vi "sutter_driver.vi"() -> ()   [LabVIEW 2016]
uses:
  <vilib>/Instr/_visa.llb/VISA Configure Serial Port (Instr).vi
panel:
  in  "Motor Poisition":dbl[][](array[numeric]) caption="Motor Poisition\nA               B"
  out "Position XYZ":dbl[](array[numeric])
  in  "Motor Select":u16(ring) items=["A"=1, "B"=2, "C"=3, "D"=4]
  in  "error in (no error)":errorcluster
  in  "stop":bool
  out "error out":errorcluster
  in  "VISA resource name":refnum<visa-resource-name>
  # "Motor Poisition\nA               B"
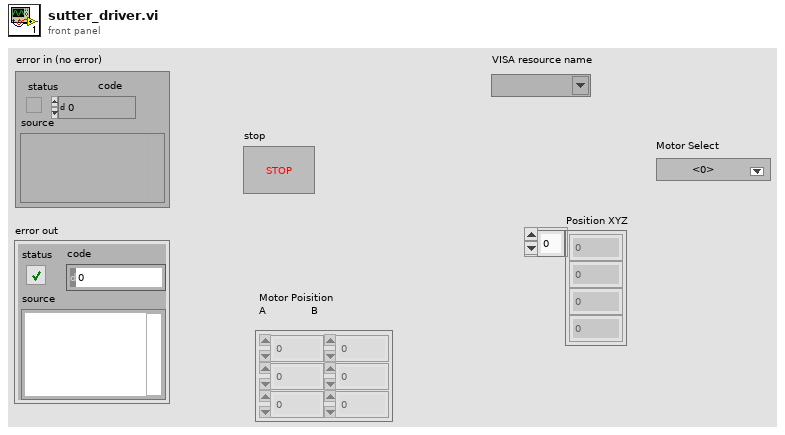
[diagram p1: front panel]
types:
  T1 = cluster{"Motor":u16, "Go Home":bool, "Position":dbl[]}
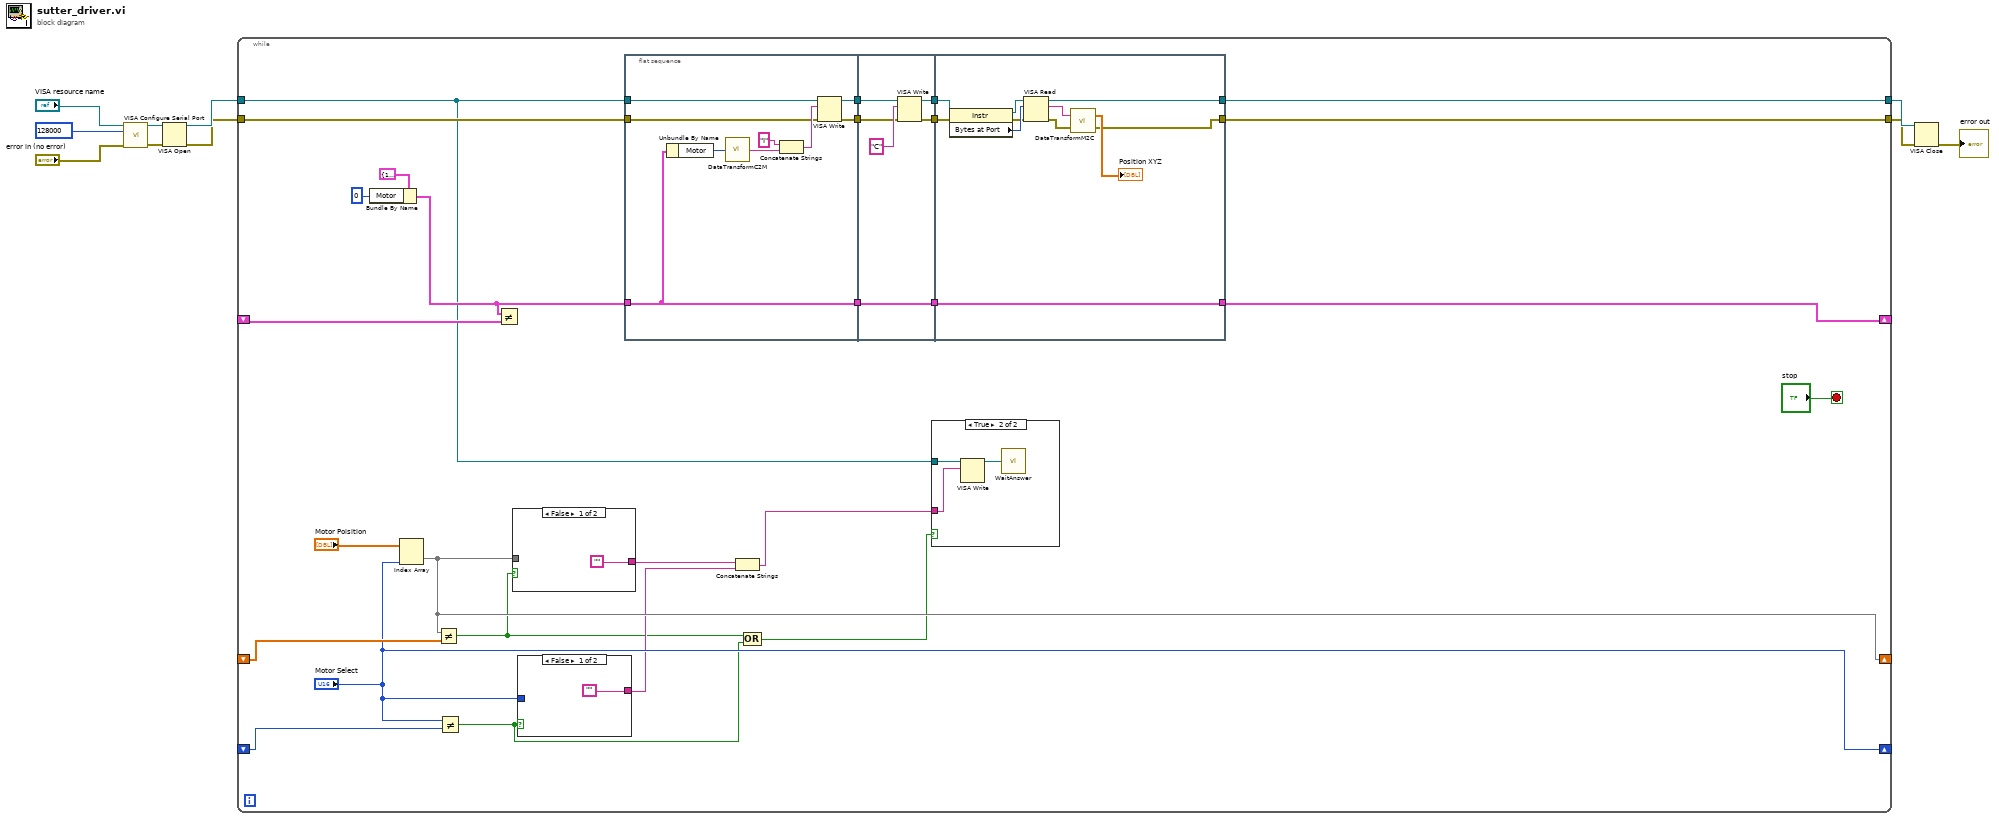
[diagram p0: block diagram]
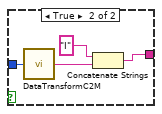
[diagram p2: hidden frame]
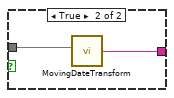
[diagram p3: hidden frame]
diagram:
  n1 = call-poly "VISA Configure Serial Port"("VISA resource name"="VISA resource name", "baud rate (9600)"=u32 128000, "error in (no error)"="error in (no error)") -> ("VISA resource name out"=w6:refnum<visa-resource-name>, "error out"=w2:errorcluster)  [unwired: 11 in]
  n2 = VISA Open(error in (no error)=w2, VISA resource name=w6) -> (VISA resource name=w5:refnum<visa-resource-name>, error out=w1:errorcluster)  [unwired: 3 in]
  n3 = while {
    tunnel: w1 -> [w36]
    tunnel: [w29] -> w7
    tunnel: w5 -> [w30]
    tunnel: [w35] -> w3
    shift-right: [w33] -> _
    shift-left: _ -> [w34]
    shift-right: [w20] -> _
    shift-left: _ -> [w28]
    shift-right: ["Motor Select"] -> _
    shift-left: _ -> [w19]
    stop <- "stop" stop-if-true
    n4 = Bundle By Name(cluster=T1 {"Motor"=1, "Go Home"=FALSE, "Position"=[0.0, 0.0, 0.0]}, "Motor"=u16 0) -> (w31:T1)
    n5 = Index Array(array="Motor Poisition", index (col)="Motor Select") -> (element=w20:dbl[])  [unwired: 1 in]
    n6 = Not Equal?(x=w20, y=w28) -> (x != y?=w13:bool)
    n7 = Not Equal?(x="Motor Select", y=w19) -> (x != y?=w11:bool)
    n8 = Not Equal?(x=w31, y=w34) -> ()  [unwired: 1 out]
    n9 = case shown="False" w13 {
      tunnel: w20 -> [_ w45]
      tunnel: ["" w44] -> w16
      frame False {
      }
      frame True {
        n10 = call "MovingDateTransform.vi"("INPUT"=w45) -> ("MOVEING COMMAND"=w44:string)  [unwired: 2 in]
      }
    }
    n11 = case shown="False" w11 {
      tunnel: "Motor Select" -> [_ w40]
      tunnel: ["" w39] -> w15
      frame False {
      }
      frame True {
        n12 = call "DataTransformC2M.vi"("input"=w40) -> ("output"=w41:string)
        n13 = Concatenate Strings("I" ("string"), w41) -> (w39:string)
      }
    }
    n14 = flat-sequence {
      tunnel: w36 -> [w51]
      tunnel: w30 -> [w54]
      tunnel: w31 -> [w46]
      tunnel: [w48] -> w24
      tunnel: [w47] -> w23
      tunnel: [w46] -> w22
      tunnel: [w59] -> w27
      tunnel: [w58] -> w26
      tunnel: [w55] -> w25
      tunnel: w24 -> [w57]
      tunnel: w23 -> [w56]
      tunnel: w22 -> [w55]
      tunnel: w27 -> [w69]
      tunnel: [w68] -> w29
      tunnel: w26 -> [w67]
      tunnel: w25 -> [w65]
      tunnel: [w65] -> w33
      tunnel: [w61] -> w35
      frame #0 {
        n15 = Unbundle By Name(w46) -> ("Motor"=w50:u16)
        n16 = call "DataTransformC2M.vi"("input"=w50) -> ("output"=w49:string)
        n17 = Concatenate Strings("I" ("string"), w49) -> (w53:string)
        n18 = VISA Write(VISA resource name=w54, write buffer=w53, error in (no error)=w51) -> (VISA resource name out=w48:refnum<visa-resource-name>, error out=w47:errorcluster)  [unwired: 1 out]
      }
      frame #1 {
        n19 = VISA Write(VISA resource name=w57, write buffer="C", error in (no error)=w56) -> (VISA resource name out=w59:refnum<visa-resource-name>, error out=w58:errorcluster)  [unwired: 1 out]
      }
      frame #2 {
        n20 = property class="Instr"(reference=w69, error in=w67) -> (reference out=w71:refnum<visa-resource-name>, error out=w66:errorcluster, "Bytes at Port"=w70:u32)
        n21 = VISA Read(VISA resource name=w71, byte count=w70, error in (no error)=w66) -> (VISA resource name out=w68:refnum<visa-resource-name>, read buffer=w64:string, error out=w63:errorcluster)  [unwired: 1 out]
        n22 = call "DataTransformM2C.vi"("ERROR IN"=w63, "MotorData"=w64) -> ("ERROR OUT"=w61:errorcluster, "Computer Data"=→"Position XYZ":dbl[])
      }
    }
    n23 = Concatenate Strings(w16, w15) -> (w14:string)
    n24 = Compound Arithmetic op=OR ("复合运算")(w13, w11) -> (w12:bool)
    n25 = case shown="True" w12 {
      tunnel: w30 -> [_ w74]
      tunnel: w14 -> [_ w73]
      frame False {
      }
      frame True {
        n26 = VISA Write(VISA resource name=w74, write buffer=w73) -> (VISA resource name out=w72:refnum<visa-resource-name>)  [unwired: 1 in, 2 out]
        n27 = call "WaitAnswer.vi"("VISA resource name out"=w72) -> ()
      }
    }
  }
  n28 = VISA Close(VISA resource name=w7, error in (no error)=w3) -> (error out=→"error out":errorcluster)
